vi "Main.vi"() -> ()   [LabVIEW 2021]
doc: "This template is for the Queued Message Handler design pattern.\n\nThe Event Handling Loop generates messages based on user interface actions.\n\nThe Message Handling Loop processes messages generated by the Event Handling Loop, or by other messages. The messages are string values, so new messages can be added easily to the Message Cases case structure in the Message Handling Loop. Each message cluster can also provide an optional value for Message Data, which is a variant that can be converted to whatever message-specific data is required."
uses:
  controls/UI Data.ctl
  support/Message Queue/Enqueue Message (Single).vi
  <vilib>/Utility/error.llb/Error Cluster From Error Code.vi
  <vilib>/ErrorRing/Error Ring.xnode
  support/Message Queue/Message Queue.lvlib
  support/User Event - Stop/User Event - Stop.lvlib
panel:
  out "Speed RPM":i32 format="%b"
  out "Data":i32
  out "hex integer string":string
  out "Write":T1
  in  "Apply Speed":bool
  out "Doing Thing":bool
  out "Speed RPM":i32(knob) scale=0.0..25.0
  in  "Speed RPM":i32(knob) min=0 max=20 scale=0.0..20.0
  in  "Max Torque Nm":i32
  out "Torque Nm":i32
  out "Torque mA":i32
  out "Max Torque mA":i32
  out "Closed Loop Available":bool
  out "Motor Initialized":bool
  out "String":string
  out "Numeric":ext
  out "Torque\n%":dbl format="%.2f"
  in  "Halt Motor":bool
  in  "ComPort":refnum<visa-resource-name>="COM1"
  out "State":string
  in  "Start Motor":bool
  in  "Exit":bool
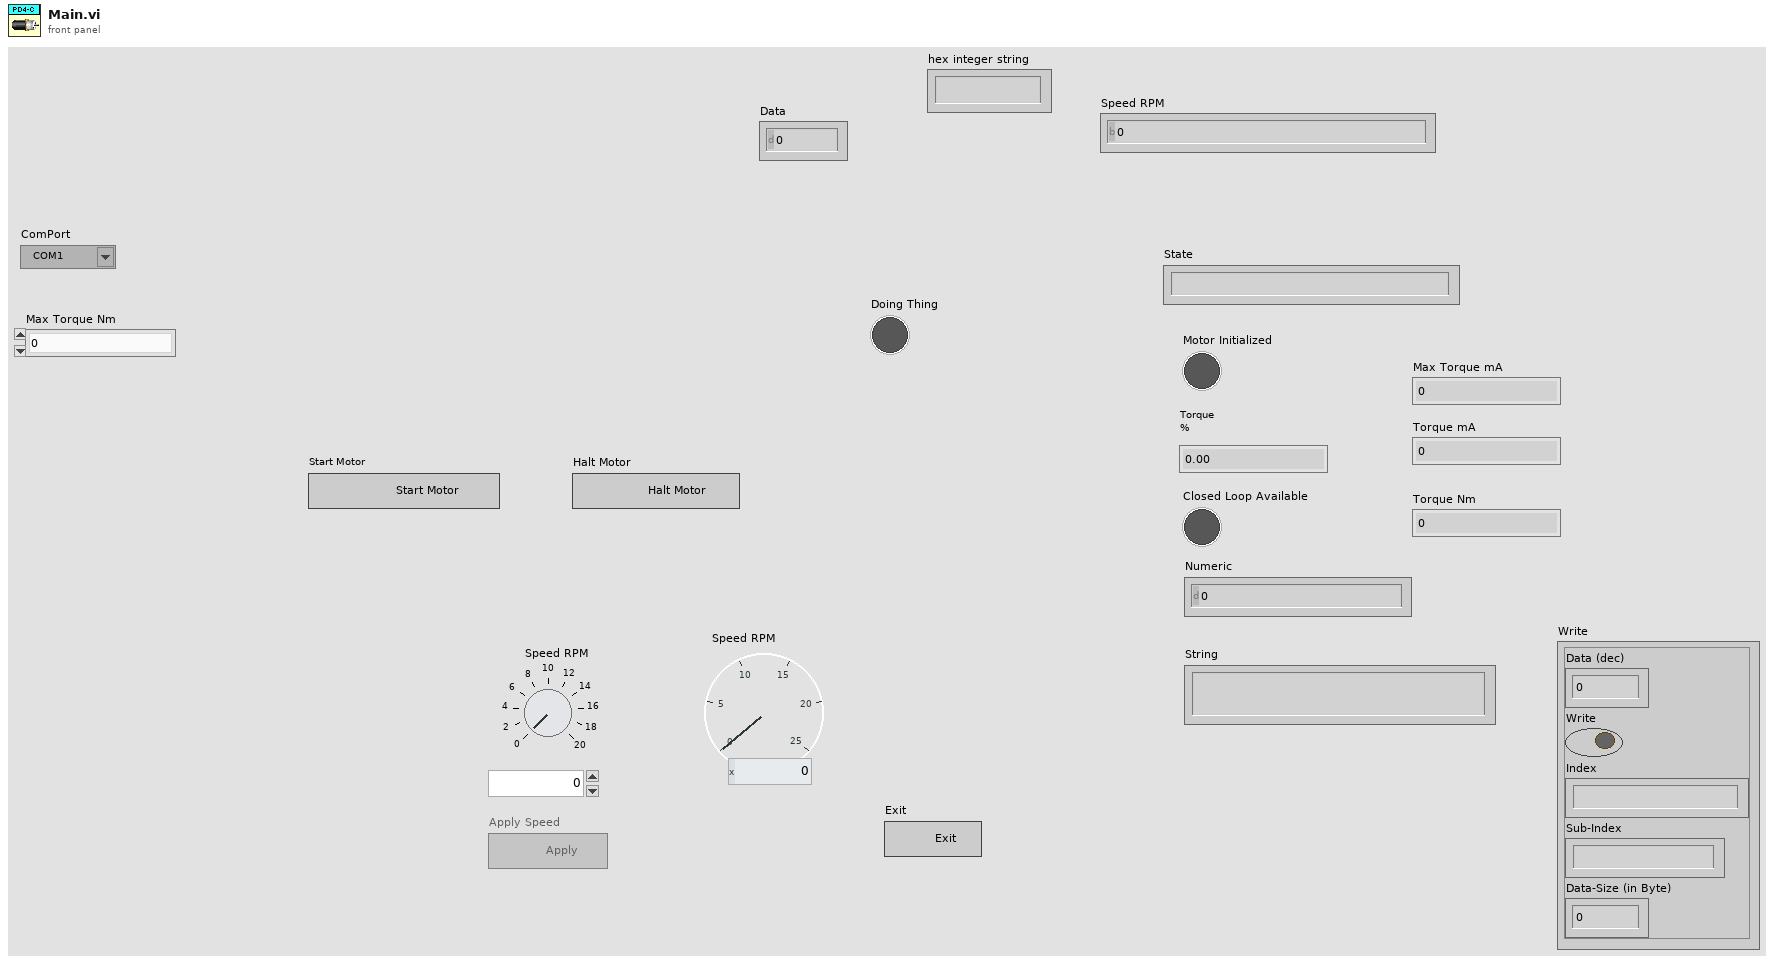
[diagram p1: front panel]
types:
  T1 = cluster{"Data (dec)":i32, "Write":bool, "Index":string, "Sub-Index":string, "Data-Size (in Byte)":u8}
  T2 = typedef "UI Data.ctl" = cluster{"Data Display Ref":refnum<vi>, "Exit Button Ref":refnum<vi>, "VISA resource name":refnum<visa-resource-name>, "Write":cluster{"Data (dec)":i32, bool, "Index":string, "Sub-Index":string, "Data-Size (in Byte)":u8}, "Next State":string, "Data":i32}
  T3 = typedef "Message Queue.lvlib/All Message Queues.ctl" = cluster{"UI":refnum<queue>}
  T4 = enum8{"Enabled", "Disabled", "Disabled and Grayed Out"}
  T5 = cluster{"Data (dec)":i32, bool, "Index":string, "Sub-Index":string, "Data-Size (in Byte)":u8}
  T6 = cluster{"Index":string, "Sub-Index":string, "Data-Size (in Byte)":u8, bool}
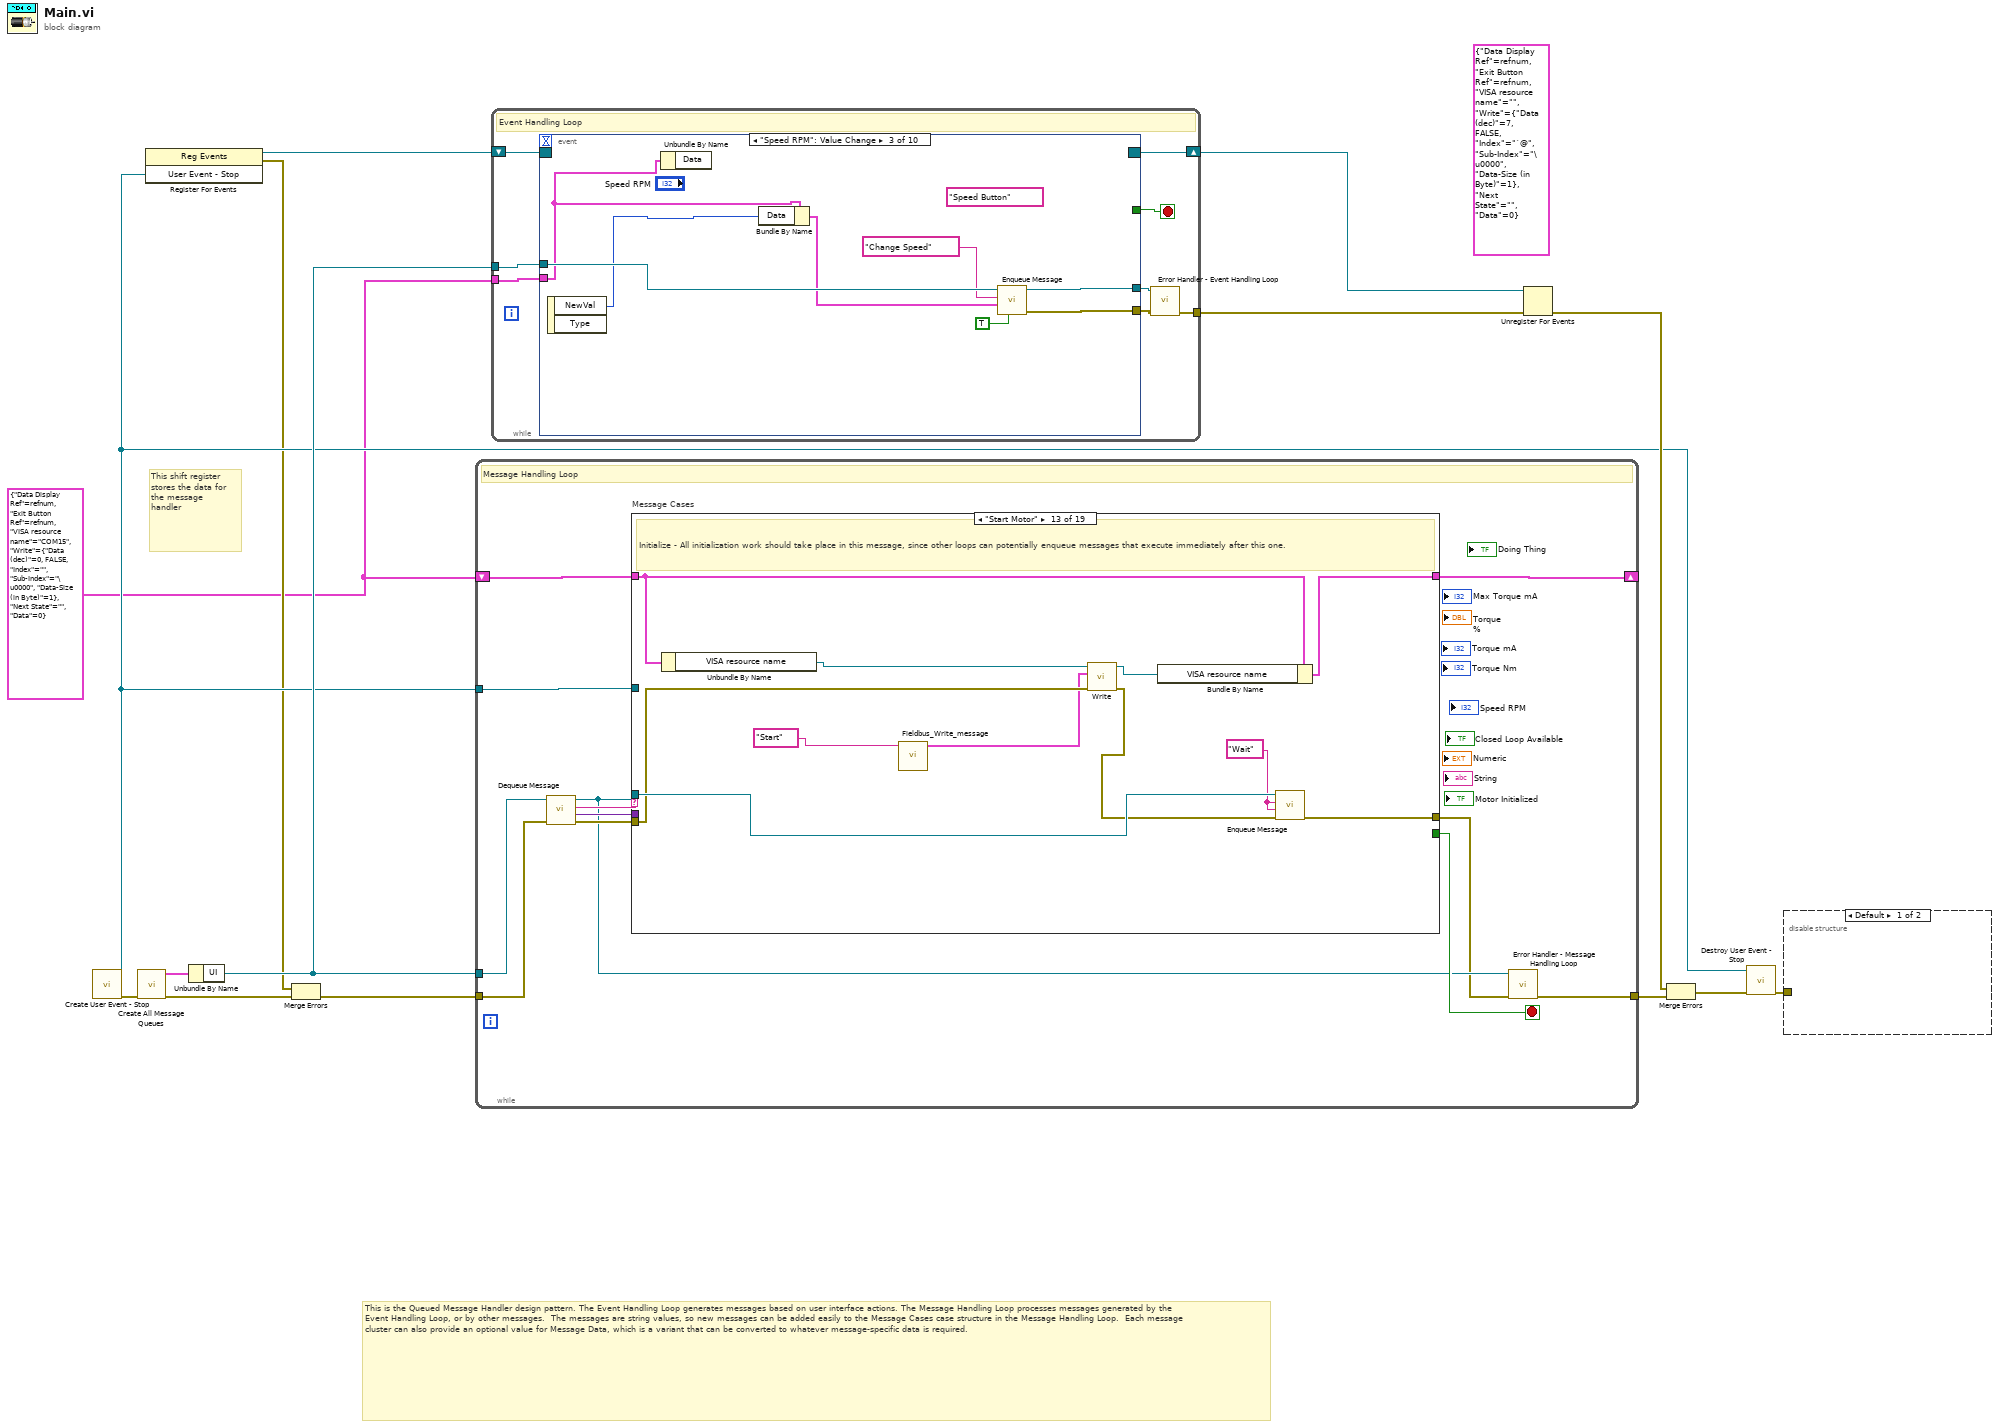
[diagram p0: block diagram]
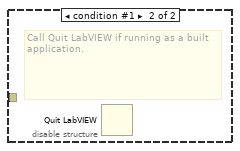
[diagram p2: hidden frame]
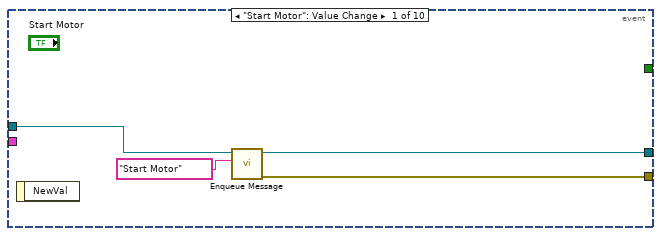
[diagram p3: hidden frame]
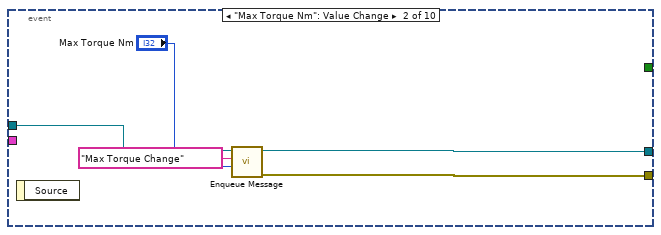
[diagram p4: hidden frame]
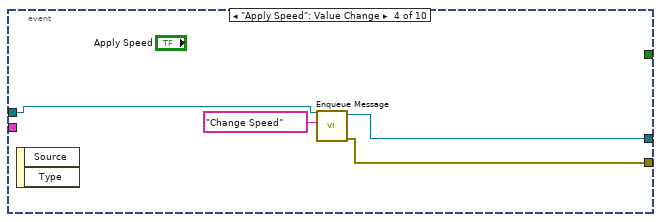
[diagram p5: hidden frame]
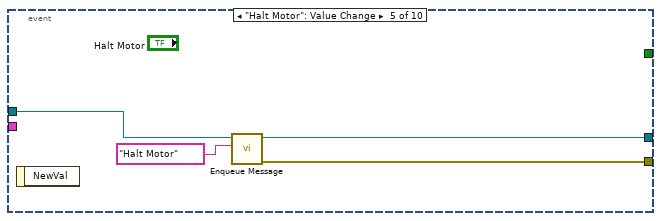
[diagram p6: hidden frame]
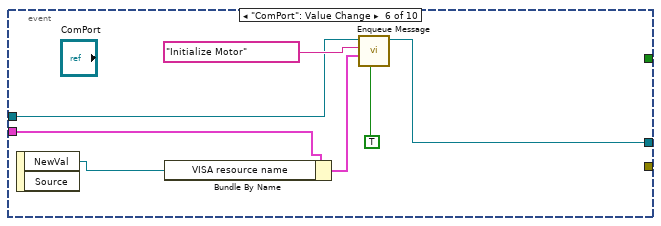
[diagram p7: hidden frame]
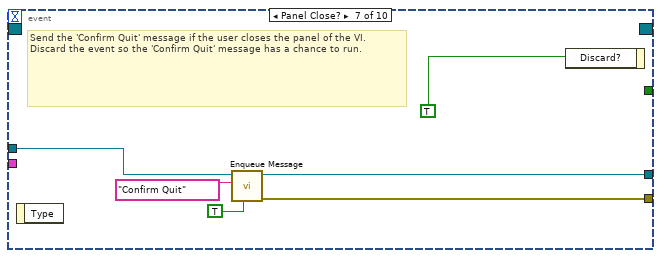
[diagram p8: hidden frame]
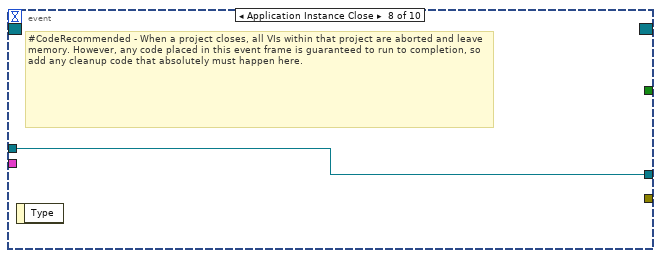
[diagram p9: hidden frame]
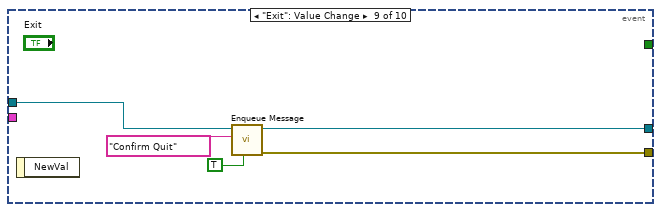
[diagram p10: hidden frame]
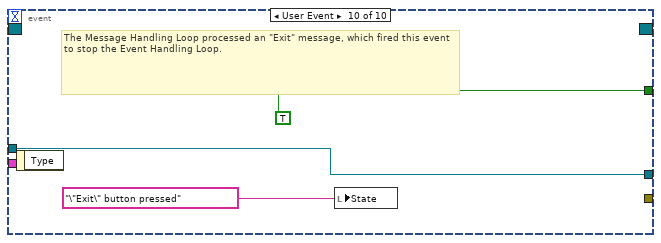
[diagram p11: hidden frame]
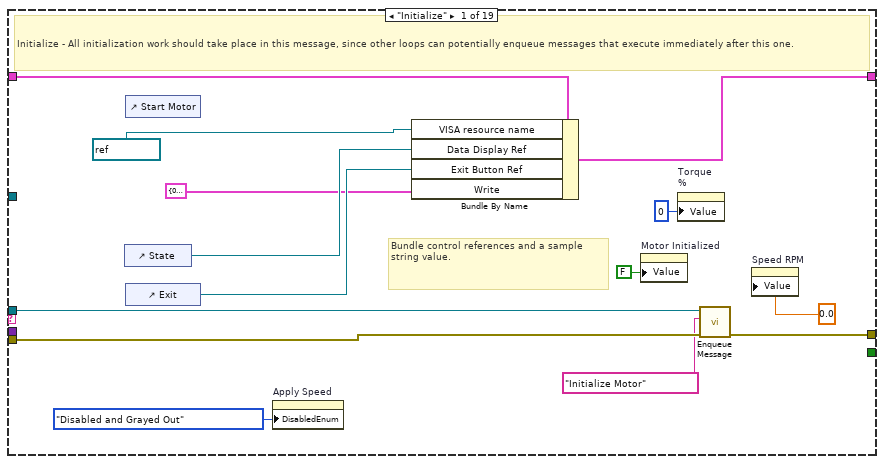
[diagram p12: hidden frame]
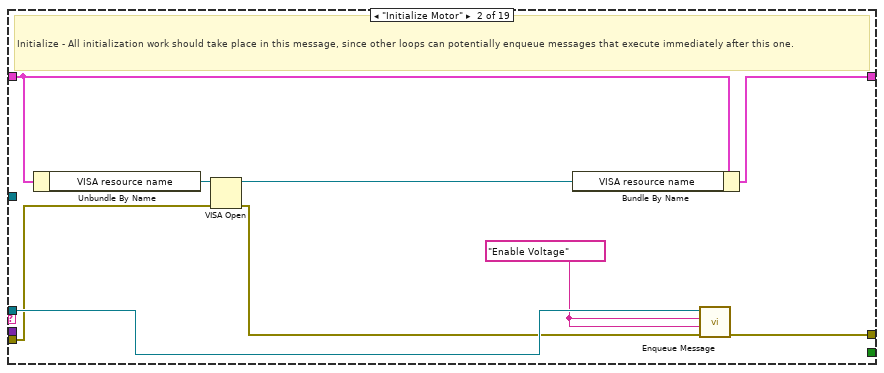
[diagram p13: hidden frame]
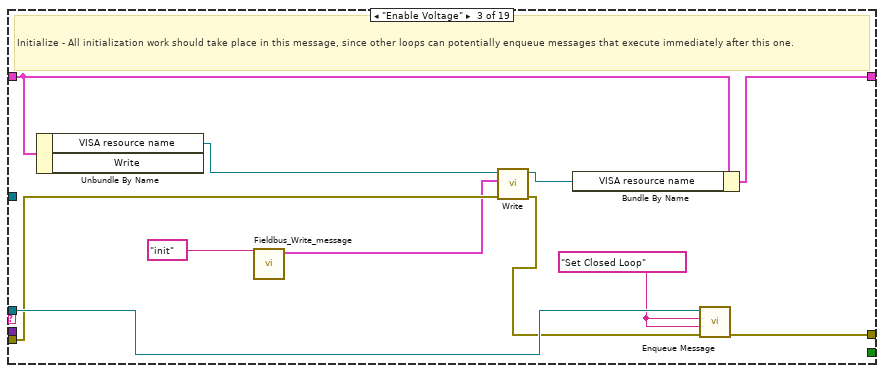
[diagram p14: hidden frame]
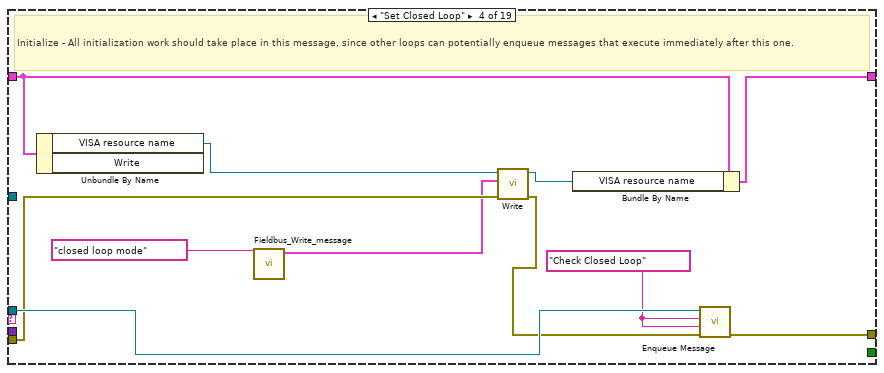
[diagram p15: hidden frame]
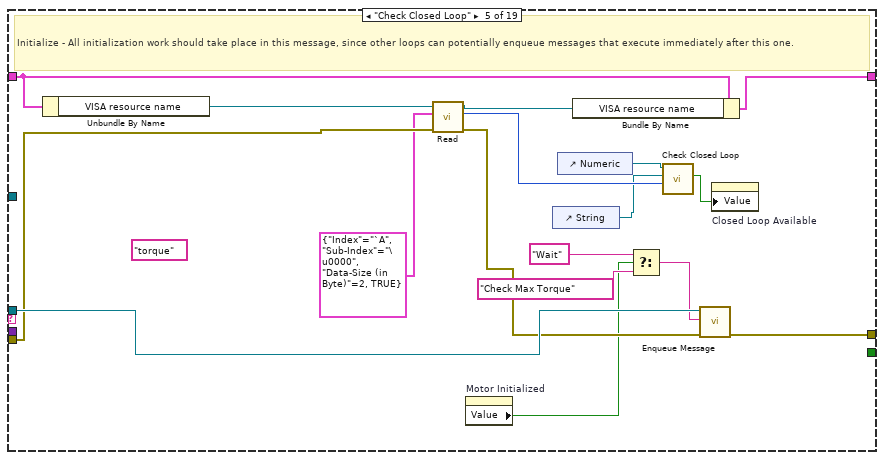
[diagram p16: hidden frame]
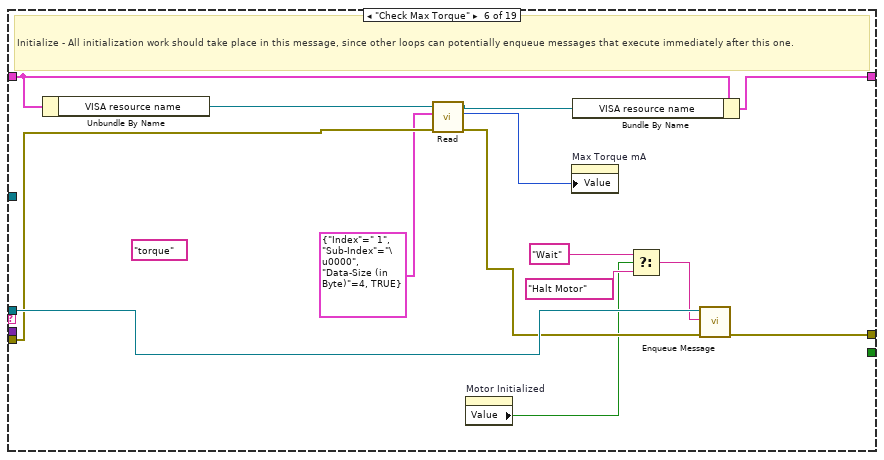
[diagram p17: hidden frame]
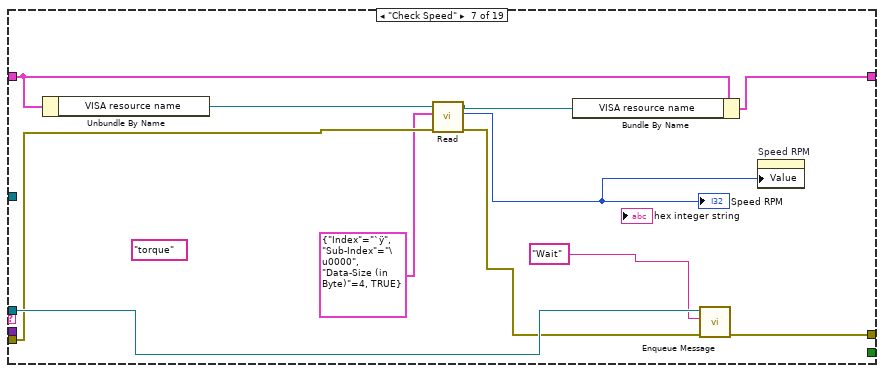
[diagram p18: hidden frame]
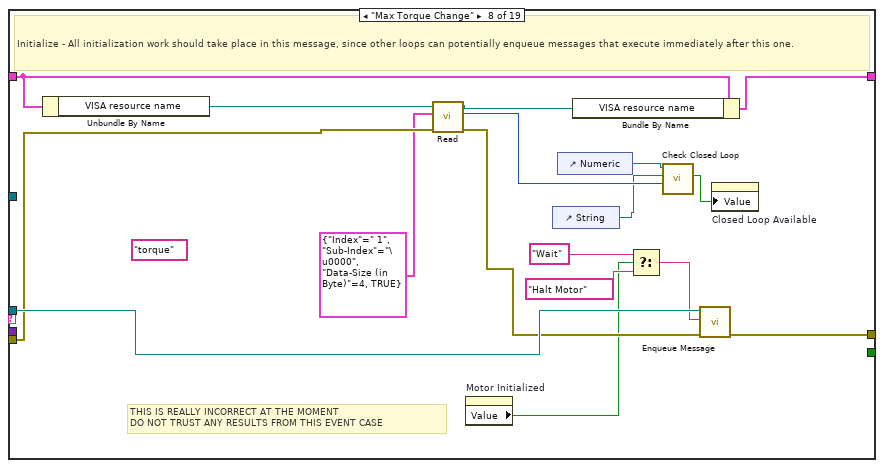
[diagram p19: hidden frame]
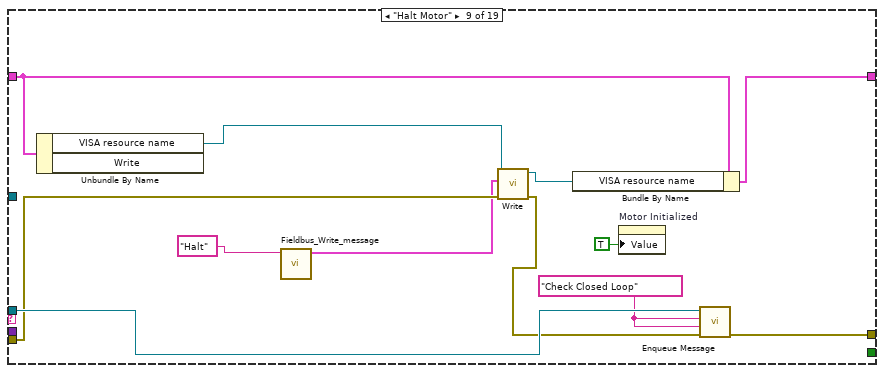
[diagram p20: hidden frame]
diagram:
  (unwired) T2 {"Data Display Ref"=refnum, "Exit Button Ref"=refnum, "VISA resource name"="", "Write"={"Data (dec)"=7, FALSE, "Index"="`@", "Sub-Index"="\u0000", "Data-Size (in Byte)"=1}, "Next State"="", "Data"=0} ("output cluster")
  w1 = T2 {"Data Display Ref"=refnum, "Exit Button Ref"=refnum, "VISA resource name"="COM15", "Write"={"Data (dec)"=0, FALSE, "Index"="", "Sub-Index"="\u0000", "Data-Size (in Byte)"=1}, "Next State"="", "Data"=0} ("Data Cluster")
  # "This is the Queued Message Handler design pattern. The Event Handling Loop generates messages based on user interface actions. The Message Handling Loop processes messages generated by the Event Handling Loop, or by other messages.  The messages are string values, so new messages can be added easily to the Message Cases case structure in the Message Handling Loop.  Each message cluster can also provide an optional value for Message Data, which is a variant that can be converted to whatever message-specific data is required."
  # "This shift register stores the data for the message handler"
  n1 = call "Create User Event - Stop.vi"() -> ("error out"=w11:errorcluster, "User Event - Stop"=w4:refnum<user-event>)  [unwired: 10 in]
  n2 = call "Create All Message Queues.vi"("error in (no error)"=w11) -> ("error out"=w15:errorcluster, "Message Queues out"=w14:T3)  [unwired: 9 in]
  n3 = register-events(w4) -> (reference out=w5:refnum<event-registration>, error out=w2:errorcluster)  [unwired: 2 in]
  n4 = Unbundle By Name "Unbundle By Name"(w14) -> ("UI"=w12:refnum<queue>)
  n5 = Merge Errors "Merge Errors"(w2, w15) -> (w3:errorcluster)
  n6 = while {
    tunnel: w12 -> [w19]
    shift-right: [w26] -> _
    shift-left: w1 -> [w27]
    tunnel: w4 -> [w24]
    tunnel: w3 -> [w23]
    tunnel: [w17] -> w13
    stop <- w25 stop-if-true
    # "Message Handling Loop"
    n7 = call "Dequeue Message.vi"("error in (no error)"=w23, "Message Queue"=w19) -> ("error out"=w22:errorcluster, "Message Data"=w20:variant, "Message"=w21:string, "dup Message Queue"=w18:refnum<queue>)  [unwired: 6 in]
    n8 = case "Message Cases" shown="\"Start Motor\"" w21 {
      selector: w21 -> [_ _ _ _ _ _ _ _ _ _ _ _ _ _ _ _ _ _ w240]
      tunnel: w18 -> [w29 w49 w60 w71 w88 w102 w113 w130 w142 w159 w164 _ w180 w193 _ _ w220 w239 _]
      tunnel: w22 -> [w40 w47 w53 w64 w85 w99 w110 w127 w135 w148 w165 w169 w173 w190 w199 w208 w212 w228 _]
      tunnel: [w41 w50 w61 w72 w89 w103 w114 w131 w143 w160 w162 w169 w181 w194 w200 w202 w222 w236 w241] -> w16
      tunnel: w27 -> [w39 w46 w59 w70 w87 w101 w112 w129 w141 w149 w166 w170 w179 w192 w201 w207 w211 w229 w242]
      tunnel: [w38 w45 w58 w69 w86 w100 w111 w128 w140 w158 w166 w170 w178 w191 w201 w207 w210 w229 w242] -> w26
      tunnel: [_ _ _ _ _ _ _ _ _ _ _ _ _ _ _ _ _ TRUE _] -> w25
      tunnel: w20 -> [_ _ _ _ _ _ _ _ _ w145 _ _ _ _ w198 w206 _ w231 _]
      tunnel: w24 -> [_ _ _ _ _ _ _ _ _ _ _ _ _ _ _ _ _ w235 _]
      frame "Initialize" {
        # "Bundle control references and a sample string value."
        # "Initialize - All initialization work should take place in this message, since other loops can potentially enqueue messages that execute immediately after this one."
        n9 = control-ref of="State"() -> (w37:refnum<vi>)
        n10 = control-ref of="Start Motor"() -> ()  [unwired: 1 out]
        n11 = control-ref of="Exit"() -> (w36:refnum<vi>)
        n12 = property on="Apply Speed" class="Bool"("DisabledEnum"=T4."Disabled and Grayed Out" ("Disabled")) -> ()  [unwired: 2 in, 2 out]
        n13 = Bundle By Name "Bundle By Name"(cluster=w39, "VISA resource name"=refnum<visa-resource-name> "COM15", "Data Display Ref"=w37, "Exit Button Ref"=w36, "Write"=T5 {"Data (dec)"=0, FALSE, "Index"="", "Sub-Index"="", "Data-Size (in Byte)"=0}) -> (w38:T2)
        n14 = property on="Motor Initialized" class="Bool (strict)"("Value"=FALSE ("Motor Initialized")) -> ()  [unwired: 2 in, 2 out]
        n15 = property on="Torque\n%" class="DigNum (strict)"("Value"=0 ("Torque\n%")) -> ()  [unwired: 2 in, 2 out]
        n16 = call-poly "Enqueue Message.vi"("error in (no error)"=w40, "Message"="Initialize Motor", "Message Queue"=w29) -> ("error out"=w41:errorcluster)  [unwired: 7 in, 1 out]
        n17 = property on="Speed RPM" class="Knob (strict)"("Value"=0.0 ("Speed RPM")) -> ()  [unwired: 2 in, 2 out]
      }
      frame "Initialize Motor" {
        w42 = "Enable Voltage" ("Message")
        # "Initialize - All initialization work should take place in this message, since other loops can potentially enqueue messages that execute immediately after this one."
        n18 = Unbundle By Name(w46) -> ("VISA resource name"=w48:refnum<visa-resource-name>)
        n19 = VISA Open(error in (no error)=w47, VISA resource name=w48) -> (VISA resource name=w44:refnum<visa-resource-name>, error out=w43:errorcluster)  [unwired: 3 in]
        n20 = Bundle By Name(cluster=w46, "VISA resource name"=w44) -> (w45:T2)
        n21 = call-poly "Enqueue Message.vi"("error in (no error)"=w43, "Message Data"=w42, "Message"=w42, "Message Queue"=w49) -> ("error out"=w50:errorcluster)  [unwired: 6 in, 1 out]
      }
      frame "Enable Voltage" {
        w55 = "Set Closed Loop" ("Message")
        # "Initialize - All initialization work should take place in this message, since other loops can potentially enqueue messages that execute immediately after this one."
        n22 = Unbundle By Name(w59) -> ("VISA resource name"=w54:refnum<visa-resource-name>)  [unwired: 1 out]
        n23 = call "Fieldbus_Write_message.vi"("Message"="init") -> ("Write"=w52:T1)  [unwired: 10 in]
        n24 = call "Write.vi"("error in"=w53, "Write"=w52, "ComPort In"=w54) -> ("error out"=w56:errorcluster, "ComPort Out"=w57:refnum<visa-resource-name>)  [unwired: 7 in]
        n25 = Bundle By Name(cluster=w59, "VISA resource name"=w57) -> (w58:T2)
        n26 = call-poly "Enqueue Message.vi"("error in (no error)"=w56, "Message Data"=w55, "Message"=w55, "Message Queue"=w60) -> ("error out"=w61:errorcluster)  [unwired: 6 in, 1 out]
      }
      frame "Set Closed Loop" {
        w66 = "Check Closed Loop" ("Message")
        # "Initialize - All initialization work should take place in this message, since other loops can potentially enqueue messages that execute immediately after this one."
        n27 = Unbundle By Name(w70) -> ("VISA resource name"=w65:refnum<visa-resource-name>)  [unwired: 1 out]
        n28 = call "Fieldbus_Write_message.vi"("Message"="closed loop mode") -> ("Write"=w63:T1)  [unwired: 10 in]
        n29 = call "Write.vi"("error in"=w64, "Write"=w63, "ComPort In"=w65) -> ("error out"=w67:errorcluster, "ComPort Out"=w68:refnum<visa-resource-name>)  [unwired: 7 in]
        n30 = Bundle By Name(cluster=w70, "VISA resource name"=w68) -> (w69:T2)
        n31 = call-poly "Enqueue Message.vi"("error in (no error)"=w67, "Message Data"=w66, "Message"=w66, "Message Queue"=w71) -> ("error out"=w72:errorcluster)  [unwired: 6 in, 1 out]
      }
      frame "Check Closed Loop" {
        (unwired) "torque" ("Message")
        # "Initialize - All initialization work should take place in this message, since other loops can potentially enqueue messages that execute immediately after this one."
        n32 = Unbundle By Name(w87) -> ("VISA resource name"=w82:refnum<visa-resource-name>)
        n33 = call "Read.vi"("error out"=w85, "Read"=T6 {"Index"="`A", "Sub-Index"="\u0000", "Data-Size (in Byte)"=2, TRUE}, "ComPort In"=w82) -> ("error out 2"=w84:errorcluster, "Answer"=w80:i32, "ComPort Out"=w81:refnum<visa-resource-name>)  [unwired: 6 in]
        n34 = property on="Motor Initialized" class="Bool (strict)"() -> ("Value"=w77:bool)  [unwired: 2 in, 2 out]
        n35 = control-ref of="String"() -> (w74:refnum<vi>)
        n36 = control-ref of="Numeric"() -> (w75:refnum<vi>)
        n37 = Bundle By Name(cluster=w87, "VISA resource name"=w81) -> (w86:T2)
        n38 = Select(t="Wait" ("Message"), s=w77, f="Check Max Torque") -> (s? t:f=w76:string)
        n39 = call "Check Closed Loop.vi"("Answer"=w80, "Str Refnum"=w74, "Digital in"=w75) -> ("Bit 0"=w73:bool)  [unwired: 8 in]
        n40 = call-poly "Enqueue Message.vi"("error in (no error)"=w84, "Message"=w76, "Message Queue"=w88) -> ("error out"=w89:errorcluster)  [unwired: 7 in, 1 out]
        n41 = property on="Closed Loop Available" class="Bool (strict)"("Value"=w73) -> ()  [unwired: 2 in, 2 out]
      }
      frame "Check Max Torque" {
        (unwired) "torque" ("Message")
        # "Initialize - All initialization work should take place in this message, since other loops can potentially enqueue messages that execute immediately after this one."
        n42 = Unbundle By Name(w101) -> ("VISA resource name"=w96:refnum<visa-resource-name>)
        n43 = call "Read.vi"("error out"=w99, "Read"=T6 {"Index"=" 1", "Sub-Index"="\u0000", "Data-Size (in Byte)"=4, TRUE}, "ComPort In"=w96) -> ("error out 2"=w98:errorcluster, "Answer"=w90:i32, "ComPort Out"=w95:refnum<visa-resource-name>)  [unwired: 6 in]
        n44 = property on="Motor Initialized" class="Bool (strict)"() -> ("Value"=w92:bool)  [unwired: 2 in, 2 out]
        n45 = property on="Max Torque mA" class="DigNum (strict)"("Value"=w90) -> ()  [unwired: 2 in, 2 out]
        n46 = Bundle By Name(cluster=w101, "VISA resource name"=w95) -> (w100:T2)
        n47 = Select(t="Wait" ("Message"), s=w92, f="Halt Motor") -> (s? t:f=w91:string)
        n48 = call-poly "Enqueue Message.vi"("error in (no error)"=w98, "Message"=w91, "Message Queue"=w102) -> ("error out"=w103:errorcluster)  [unwired: 7 in, 1 out]
      }
      frame "Check Speed" {
        (unwired) "torque" ("Message")
        n49 = Unbundle By Name(w112) -> ("VISA resource name"=w107:refnum<visa-resource-name>)
        n50 = call "Read.vi"("error out"=w110, "Read"=T6 {"Index"="`ÿ", "Sub-Index"="\u0000", "Data-Size (in Byte)"=4, TRUE}, "ComPort In"=w107) -> ("error out 2"=w109:errorcluster, "Answer"=w104:i32, "ComPort Out"=w106:refnum<visa-resource-name>)  [unwired: 6 in]
        "Speed RPM" <- w104
        n51 = Bundle By Name(cluster=w112, "VISA resource name"=w106) -> (w111:T2)
        n52 = call-poly "Enqueue Message.vi"("error in (no error)"=w109, "Message"="Wait", "Message Queue"=w113) -> ("error out"=w114:errorcluster)  [unwired: 7 in, 1 out]
        n53 = property on="Speed RPM" class="Knob (strict)"("Value"=w104) -> ()  [unwired: 2 in, 2 out]
      }
      frame "Max Torque Change" {
        (unwired) "torque" ("Message")
        # "THIS IS REALLY INCORRECT AT THE MOMENT\nDO NOT TRUST ANY RESULTS FROM THIS EVENT CASE"
        # "Initialize - All initialization work should take place in this message, since other loops can potentially enqueue messages that execute immediately after this one."
        n54 = Unbundle By Name(w129) -> ("VISA resource name"=w124:refnum<visa-resource-name>)
        n55 = call "Read.vi"("error out"=w127, "Read"=T6 {"Index"=" 1", "Sub-Index"="\u0000", "Data-Size (in Byte)"=4, TRUE}, "ComPort In"=w124) -> ("error out 2"=w126:errorcluster, "Answer"=w122:i32, "ComPort Out"=w123:refnum<visa-resource-name>)  [unwired: 6 in]
        n56 = property on="Motor Initialized" class="Bool (strict)"() -> ("Value"=w119:bool)  [unwired: 2 in, 2 out]
        n57 = control-ref of="String"() -> (w116:refnum<vi>)
        n58 = control-ref of="Numeric"() -> (w117:refnum<vi>)
        n59 = Bundle By Name(cluster=w129, "VISA resource name"=w123) -> (w128:T2)
        n60 = Select(t="Wait" ("Message"), s=w119, f="Halt Motor") -> (s? t:f=w118:string)
        n61 = call "Check Closed Loop.vi"("Answer"=w122, "Str Refnum"=w116, "Digital in"=w117) -> ("Bit 0"=w115:bool)  [unwired: 8 in]
        n62 = call-poly "Enqueue Message.vi"("error in (no error)"=w126, "Message"=w118, "Message Queue"=w130) -> ("error out"=w131:errorcluster)  [unwired: 7 in, 1 out]
        n63 = property on="Closed Loop Available" class="Bool (strict)"("Value"=w115) -> ()  [unwired: 2 in, 2 out]
      }
      frame "Halt Motor" {
        w137 = "Check Closed Loop" ("Message")
        n64 = Unbundle By Name(w141) -> ("VISA resource name"=w136:refnum<visa-resource-name>)  [unwired: 1 out]
        n65 = call "Fieldbus_Write_message.vi"("Message"="Halt") -> ("Write"=w133:T1)  [unwired: 10 in]
        n66 = call "Write.vi"("error in"=w135, "Write"=w133, "ComPort In"=w136) -> ("error out"=w138:errorcluster, "ComPort Out"=w139:refnum<visa-resource-name>)  [unwired: 7 in]
        n67 = Bundle By Name(cluster=w141, "VISA resource name"=w139) -> (w140:T2)
        n68 = property on="Motor Initialized" class="Bool (strict)"("Value"=TRUE ("Motor Initialized")) -> ()  [unwired: 2 in, 2 out]
        n69 = call-poly "Enqueue Message.vi"("error in (no error)"=w138, "Message Data"=w137, "Message"=w137, "Message Queue"=w142) -> ("error out"=w143:errorcluster)  [unwired: 6 in, 1 out]
      }
      frame "Change Speed" {
        w155 = "Check Speed" ("Message")
        n70 = Variant To Data(error in=w148, type=w149, Variant=w145) -> (data=w146:T2, error out=w147:errorcluster)
        n71 = Unbundle By Name(w146) -> ("Data"=w144:i32)
        "Data" <- w144
        n72 = Unbundle By Name(w149) -> ("VISA resource name"=w154:refnum<visa-resource-name>)
        n73 = call "Fieldbus_Write_message.vi"("Data"=w144, "Message"="change speed") -> ("Write"=w152:T1)  [unwired: 9 in]
        "Write" <- w152
        n74 = property on="Apply Speed" class="Bool"("DisabledEnum"=T4."Disabled and Grayed Out" ("Disabled")) -> ()  [unwired: 2 in, 2 out]
        n75 = disable-structure shown="Enabled" {
          frame Disabled {
            n76 = property on="Speed RPM" class="Knob (strict)" props=["Value"]() -> ()  [unwired: 3 in, 2 out]
          }
          frame Enabled {
          }
        }
        n77 = call "Write.vi"("error in"=w147, "Write"=w152, "ComPort In"=w154) -> ("error out"=w156:errorcluster, "ComPort Out"=w157:refnum<visa-resource-name>)  [unwired: 7 in]
        n78 = Bundle By Name(cluster=w149, "VISA resource name"=w157) -> (w158:T2)
        n79 = property on="Doing Thing" class="Bool (strict)"("Value"=TRUE ("Doing Thing")) -> ()  [unwired: 2 in, 2 out]
        n80 = call-poly "Enqueue Message.vi"("error in (no error)"=w156, "Message Data"=w155, "Message"=w155, "Message Queue"=w159) -> ("error out"=w160:errorcluster)  [unwired: 6 in, 1 out]
      }
      frame "Speed Button" {
        # "Initialize - All initialization work should take place in this message, since other loops can potentially enqueue messages that execute immediately after this one."
        n81 = property on="Apply Speed" class="Bool"("DisabledEnum"=T4."Enabled" ("Disabled")) -> ()  [unwired: 2 in, 2 out]
        n82 = property on="Doing Thing" class="Bool (strict)"("Value"=TRUE ("Doing Thing")) -> ()  [unwired: 2 in, 2 out]
        n83 = call-poly "Enqueue Message.vi"("error in (no error)"=w165, "Message"="Wait", "Message Queue"=w164) -> ("error out"=w162:errorcluster)  [unwired: 7 in, 1 out]
      }
      frame "Wait" {
        # "Initialize - All initialization work should take place in this message, since other loops can potentially enqueue messages that execute immediately after this one."
        n84 = property on="Doing Thing" class="Bool (strict)"("Value"=FALSE ("Doing Thing")) -> ()  [unwired: 2 in, 2 out]
      }
      frame "Start Motor" {
        w175 = "Wait" ("Message")
        # "Initialize - All initialization work should take place in this message, since other loops can potentially enqueue messages that execute immediately after this one."
        n85 = Unbundle By Name(w179) -> ("VISA resource name"=w174:refnum<visa-resource-name>)
        n86 = call "Fieldbus_Write_message.vi"("Message"="Start") -> ("Write"=w171:T1)  [unwired: 10 in]
        n87 = call "Write.vi"("error in"=w173, "Write"=w171, "ComPort In"=w174) -> ("error out"=w176:errorcluster, "ComPort Out"=w177:refnum<visa-resource-name>)  [unwired: 7 in]
        n88 = Bundle By Name(cluster=w179, "VISA resource name"=w177) -> (w178:T2)
        n89 = call-poly "Enqueue Message.vi"("error in (no error)"=w176, "Message Data"=w175, "Message"=w175, "Message Queue"=w180) -> ("error out"=w181:errorcluster)  [unwired: 6 in, 1 out]
      }
      frame "Get Torque" {
        (unwired) "torque" ("Message")
        # "Initialize - All initialization work should take place in this message, since other loops can potentially enqueue messages that execute immediately after this one."
        n90 = Unbundle By Name(w192) -> ("VISA resource name"=w187:refnum<visa-resource-name>)
        n91 = call "Read.vi"("error out"=w190, "Read"=T6 {"Index"="`w", "Sub-Index"="\u0000", "Data-Size (in Byte)"=2, TRUE}, "ComPort In"=w187) -> ("error out 2"=w189:errorcluster, "Answer"=w185:i32, "ComPort Out"=w186:refnum<visa-resource-name>)  [unwired: 6 in]
        n92 = Divide(x=w185, y=1000) -> (x/y=w182:dbl)
        n93 = Bundle By Name(cluster=w192, "VISA resource name"=w186) -> (w191:T2)
        n94 = property on="Torque\n%" class="DigNum (strict)"("Value"=w182) -> ()  [unwired: 2 in, 2 out]
        n95 = call-poly "Enqueue Message.vi"("error in (no error)"=w189, "Message"="Get Torque", "Message Queue"=w193) -> ("error out"=w194:errorcluster)  [unwired: 7 in, 1 out]
      }
      frame "Update Display" {
        # "#CodeRecommended - If you wish to decouple the Message Handling Loop from your user interface, consider creating User Events (like the \"Stop\" event in this VI) to message the Event Handling Loop whenever the user interface needs updating."
        # "Update Display - Convert the message data to a string to display in the Data Display indicator."
        n96 = Variant To Data(error in=w199, type="", Variant=w198) -> (data=→"State":string, error out=w196:errorcluster)
        n97 = Merge Errors(w196) -> (w200:errorcluster)
      }
      frame "Error" {
        # "#CodeRecommended - If you ever change the name of this \"Error\" message, you'll need to update the name in the Check Loop Error.vi as well."
        # "#CodeRecommended - Consider creating a system for logging errors in some way. These errors are for notification purposes only. Handling of specific errors should be performed in the message frames that generated the error."
        # "Error - Display an error dialog. This message is sent by the \"Error Handler\" VIs at the end of other loops in this application."
        n98 = Variant To Data(error in=w208, type=errorcluster {"status"=FALSE, "code"=0, "source"=""} ("error constant"), Variant=w206) -> (data=w204:errorcluster, error out=w203:errorcluster)
        n99 = call <vilib>:"Simple Error Handler.vi"("error in (no error)"=w204) -> ()  [unwired: 4 in, 5 out]
        n100 = Merge Errors(w203) -> (w202:errorcluster)
      }
      frame "Confirm Quit" {
        # "#CodeNeeded - If you want to provide an \"Are you sure\" dialog (or some other notification) before the application exits, place that code here. This message is typically sent from a Panel Close? event."
        # "Confirm Quit - Message that can confirm whether or not the user wants to exit the application."
        n101 = Unbundle By Name(w211) -> ("VISA resource name"=w216:refnum<visa-resource-name>)  [unwired: 1 out]
        n102 = call "Fieldbus_Write_message.vi"("Message"="Halt") -> ("Write"=w214:T1)  [unwired: 10 in]
        n103 = call "Write.vi"("error in"=w212, "Write"=w214, "ComPort In"=w216) -> ("error out"=w213:errorcluster, "ComPort Out"=w217:refnum<visa-resource-name>)  [unwired: 7 in]
        n104 = Bundle By Name(cluster=w211, "VISA resource name"=w217) -> (w210:T2)
        n105 = call-poly "Enqueue Message.vi"("Priority Message? (F)"=TRUE, "error in (no error)"=w212, "Message"="Exit", "Message Queue"=w220) -> ("error out"=w221:errorcluster)  [unwired: 6 in, 1 out]
        n106 = property on="Motor Initialized" class="Bool (strict)"("Value"=FALSE ("Motor Initialized")) -> ()  [unwired: 2 in, 2 out]
        n107 = Merge Errors(w213, w221) -> (w222:errorcluster)
      }
      frame "Exit" {
        # "Stop the VI"
        # "Release the message queue reference"
        # "#CodeNeeded - Add any required cleanup code here. Note that if 'Exit' was called as a result of an error, an error dialog will be displayed. Add any custom error handling for an 'Exit' condition here as well."
        # "Exit - Exit the application."
        n108 = Unbundle By Name(w229) -> ("VISA resource name"=w230:refnum<visa-resource-name>)
        n109 = Variant To Data(type=errorcluster {"status"=FALSE, "code"=0, "source"=""} ("error constant"), Variant=w231) -> (data=w232:errorcluster)  [unwired: 1 in, 1 out]
        n110 = call <vilib>:"Simple Error Handler.vi"("error in (no error)"=w232) -> ()  [unwired: 4 in, 5 out]
        n111 = VISA Close(VISA resource name=w230, error in (no error)=w228) -> (error out=w227:errorcluster)
        n112 = call "Fire User Event - Stop.vi"("User Event - Stop"=w235) -> ("error out"=w234:errorcluster)  [unwired: 10 in]
        n113 = Release Queue(queue=w239, error in (no error)=w227) -> (error out=w237:errorcluster)  [unwired: 1 in, 2 out]
        n114 = Merge Errors(w234, w237) -> (w236:errorcluster)
        n115 = property on="Max Torque mA" class="DigNum (strict)"("Value"=0 ("Max Torque mA")) -> ()  [unwired: 2 in, 2 out]
        n116 = property on="String" class="Str"("Value"="0" ("String")) -> ()  [unwired: 2 in, 2 out]
        n117 = property on="Numeric" class="DigNum (strict)"("Value"=ext 0.0 ("Numeric")) -> ()  [unwired: 2 in, 2 out]
        n118 = property on="Motor Initialized" class="Bool (strict)"("Value"=FALSE ("Motor Initialized")) -> ()  [unwired: 2 in, 2 out]
      }
      frame Default {
        # "'Default' case only runs if there is a message that isn't defined in any of the other cases.  Output a programming error."
        n119 = xnode "Error Ring"("parameter 0"=w240) -> ("error out"=w241:errorcluster)
      }
    }
    n120 = call "Error Handler - Message Handling Loop.vi"("error in (no error)"=w16, "Message Queue"=w18) -> ("dup error in"=w17:errorcluster)  [unwired: 8 in, 1 out]
  }
  n121 = while {
    tunnel: w12 -> [w257]
    shift-right: [w255] -> w8
    shift-left: w5 -> [w256]
    tunnel: [w251] -> w6
    tunnel: w1 -> [w250]
    stop <- w253 stop-if-true
    # "Event Handling Loop"
    n122 = event shown="[2] \"Speed RPM\": Value Change" {
      selector: w256 -> [_ _ _ _ _ _ _ _ _ _]
      dyn-events: [_ _ _ _ _ _ _ _ _ _] -> w255
      timeout: _ -> [_ _ _ _ _ _ _ _ _ _]
      tunnel: [_ _ _ _ _ _ _ _ _ TRUE ("Discard?")] -> w253
      tunnel: w257 -> [w261 w266 w274 w277 w282 w288 w294 w296 w301 w304]
      tunnel: [w258 w264 w272 w275 w279 _ w293 _ w300 _] -> w254
      tunnel: [w260 w265 w273 w276 w281 w287 w292 w296 w299 w304] -> w252
      tunnel: w250 -> [_ _ w268 _ _ w283 _ _ _ _]
      event "Start Motor": Value Change {
        n123 = event-data() -> ()  [unwired: 1 in, 1 out]
        n124 = call-poly "Enqueue Message.vi"("Message"="Start Motor", "Message Queue"=w261) -> ("error out"=w258:errorcluster, "dup Message Queue"=w260:refnum<queue>)  [unwired: 8 in]
      }
      event "Max Torque Nm": Value Change {
        n125 = event-data() -> ()  [unwired: 1 in, 1 out]
        n126 = call-poly "Enqueue Message.vi"("Message Data"="Max Torque Nm", "Message"="Max Torque Change", "Message Queue"=w266) -> ("error out"=w264:errorcluster, "dup Message Queue"=w265:refnum<queue>)  [unwired: 7 in]
      }
      event "Speed RPM": Value Change {
        (unwired) "Speed Button" ("Message")
        n127 = event-data() -> ("NewVal"=w267:i32)  [unwired: 1 in, 1 out]
        n128 = Unbundle By Name(w268) -> ()  [unwired: 1 out]
        n129 = Bundle By Name(cluster=w268, "Data"=w267) -> (w271:T2)
        n130 = call-poly "Enqueue Message.vi"("Priority Message? (F)"=TRUE, "Message Data"=w271, "Message"="Change Speed", "Message Queue"=w274) -> ("error out"=w272:errorcluster, "dup Message Queue"=w273:refnum<queue>)  [unwired: 6 in]
      }
      event "Apply Speed": Value Change {
        n131 = event-data() -> ()  [unwired: 1 in, 2 out]
        n132 = call-poly "Enqueue Message.vi"("Message"="Change Speed", "Message Queue"=w277) -> ("error out"=w275:errorcluster, "dup Message Queue"=w276:refnum<queue>)  [unwired: 8 in]
      }
      event "Halt Motor": Value Change {
        n133 = event-data() -> ()  [unwired: 1 in, 1 out]
        n134 = call-poly "Enqueue Message.vi"("Message"="Halt Motor", "Message Queue"=w282) -> ("error out"=w279:errorcluster, "dup Message Queue"=w281:refnum<queue>)  [unwired: 8 in]
      }
      event "ComPort": Value Change {
        n135 = event-data() -> ("NewVal"=w285:refnum<visa-resource-name>)  [unwired: 1 in, 1 out]
        n136 = Bundle By Name(cluster=w283, "VISA resource name"=w285) -> (w284:T2)
        n137 = call-poly "Enqueue Message.vi"("Priority Message? (F)"=TRUE, "Message Data"=w284, "Message"="Initialize Motor", "Message Queue"=w288) -> ("dup Message Queue"=w287:refnum<queue>)  [unwired: 6 in, 1 out]
      }
      event Panel Close? {
        # "Send the 'Confirm Quit' message if the user closes the panel of the VI. Discard the event so the 'Confirm Quit' message has a chance to run."
        n138 = event-data() -> ()  [unwired: 1 in, 1 out]
        n139 = call-poly "Enqueue Message.vi"("Priority Message? (F)"=TRUE, "Message"="Confirm Quit", "Message Queue"=w294) -> ("error out"=w293:errorcluster, "dup Message Queue"=w292:refnum<queue>)  [unwired: 7 in]
        n140 = event-data("Discard?"=TRUE) -> ()  [unwired: 1 in, 1 out]
      }
      event Application Instance Close {
        # "#CodeRecommended - When a project closes, all VIs within that project are aborted and leave memory. However, any code placed in this event frame is guaranteed to run to completion, so add any cleanup code that absolutely must happen here."
        n141 = event-data() -> ()  [unwired: 1 in, 1 out]
      }
      event "Exit": Value Change {
        n142 = event-data() -> ()  [unwired: 1 in, 1 out]
        n143 = call-poly "Enqueue Message.vi"("Priority Message? (F)"=TRUE, "Message"="Confirm Quit", "Message Queue"=w301) -> ("error out"=w300:errorcluster, "dup Message Queue"=w299:refnum<queue>)  [unwired: 7 in]
      }
      event User Event {
        # "The Message Handling Loop processed an \"Exit\" message, which fired this event to stop the Event Handling Loop."
        n144 = event-data() -> ()  [unwired: 1 in, 1 out]
        n145 = local write "State"("\"Exit\" button pressed" ("VI Stopped")) -> ()
      }
    }
    n146 = call "Error Handler - Event Handling Loop.vi"("error in (no error)"=w254, "Message Queue"=w252) -> ("dup error in"=w251:errorcluster)  [unwired: 8 in, 1 out]
  }
  n147 = Unregister For Events(event registration refnum=w8, error in=w6) -> (error out=w9:errorcluster)
  n148 = Merge Errors(w9, w13) -> (w10:errorcluster)
  n149 = call "Destroy User Event - Stop.vi"("error in (no error)"=w10, "User Event - Stop"=w4) -> ("error out"=w7:errorcluster)  [unwired: 9 in]
  n150 = disable-structure shown="Default" {
    disable-tunnel: w7 -> [_ _]
    frame condition #0 (active) {
    }
    frame condition #1 {
      # "Call Quit LabVIEW if running as a built application."
      n151 = Quit LabVIEW() -> ()  [unwired: 1 in]
    }
  }
